vi "Get Scaling Equation.vi"(0 "session in":refnum<k21>, 5 "physical channel":refnum<k21>="$DefaultPhysChans", 11 "error in (no error)":errorcluster) -> (4 "session out":refnum<k21>, 6 "physical channel out":refnum<k21>, 8 "equation":string, 15 "error out":errorcluster)   [LabVIEW 2020, in "SLSC.lvlib"]
doc: "Gets a scaling equation from a user-defined scale."
uses:
  <vilib>/SLSC/SLSC.lvlib
  nislsclvapi.dll
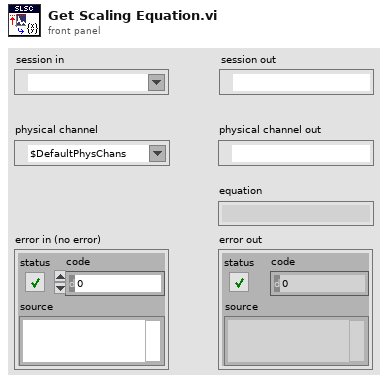
[diagram p1: front panel]
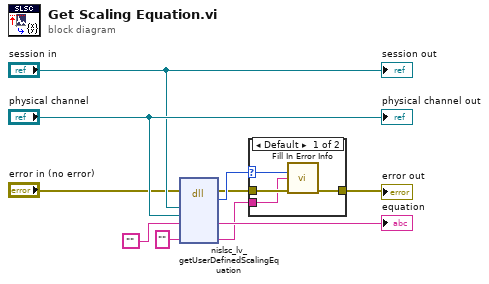
[diagram p0: block diagram]
diagram:
  n1 = dll-call lib="nislsclvapi.*" fn="nislsc_lv_getUserDefinedScalingEquation"(error in="error in (no error)", "session"="session in", "physical channel"="physical channel", "equation"="", "extendedErrorInfo"="") -> (error out=w3:errorcluster, "return type"=w4:i32, "equation"=→"equation":string, "extendedErrorInfo"=w1:string)  [unwired: 6 in, 1 out]
  n2 = case shown="Default" w4 {
    selector: w4 -> [w14 _]
    tunnel: w1 -> [w12 _]
    tunnel: w3 -> [w13 w15]
    tunnel: [w11 w15] -> w2
    frame Default {
      n3 = call <vilib>:"Fill In Error Info.vi"("status code"=w14, "extended error info"=w12, "error in"=w13) -> ("error out"=w11:errorcluster)  [unwired: 12 in]
    }
    frame 0 {
    }
  }
  "error out" <- w2
  "session out" <- "session in"
  "physical channel out" <- "physical channel"
